vi "TUNA parse navigation string.vi"(2 "Header":string="T", 3 "Nav String":string="$,A,43,13,230,B,10,20,120,C,10,10,330,D,14,36,110,T,08,12,234\r") -> (0 "Valid?":bool, 1 "Output GPS":cluster{"X POS":i32, "Y POS":i32, "HEADING":dbl})   [LabVIEW 2014]
doc: "This VI will parse the Tug navigation string for the Tug letters, A for example, and the time, T. It returns a cluster with the Tug / Time and three values as decimals."
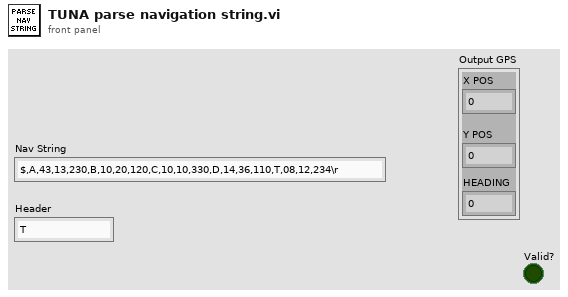
[diagram p1: front panel]
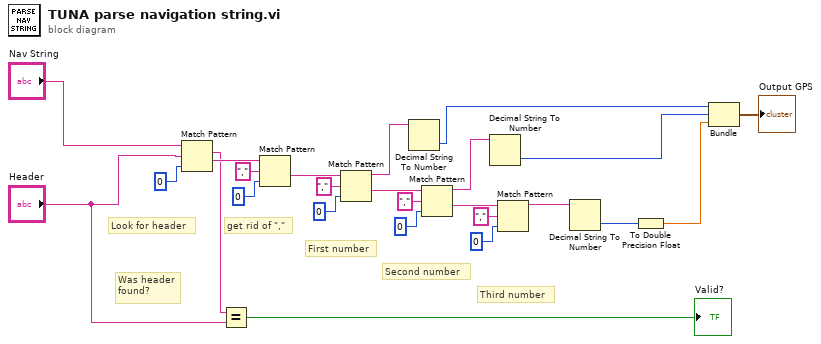
[diagram p0: block diagram]
diagram:
  # "Was header\nfound?"
  # "Third number"
  # "Second number"
  # "First number"
  # "get rid of \",\""
  # "Look for header"
  n1 = Match Pattern(string="Nav String", regular expression="Header", offset (0)=0) -> (match substring=w8:string, after substring=w10:string)  [unwired: 2 out]
  n2 = Equal?(x=w8, y="Header") -> (x = y?=→"Valid?":bool)
  n3 = Match Pattern(string=w10, regular expression=",", offset (0)=0) -> (after substring=w11:string)  [unwired: 3 out]
  n4 = Match Pattern(string=w11, regular expression=",", offset (0)=0) -> (before substring=w22:string, after substring=w18:string)  [unwired: 2 out]
  n5 = Decimal String To Number(string=w22) -> (number=w4:i32)  [unwired: 2 in, 1 out]
  n6 = Match Pattern(string=w18, regular expression=",", offset (0)=0) -> (before substring=w19:string, after substring=w14:string)  [unwired: 2 out]
  n7 = Decimal String To Number(string=w19) -> (number=w3:i32)  [unwired: 2 in, 1 out]
  n8 = Match Pattern(string=w14, regular expression=",", offset (0)=0) -> (before substring=w15:string)  [unwired: 3 out]
  n9 = Decimal String To Number(string=w15) -> (number=w2:i32)  [unwired: 2 in, 1 out]
  n10 = To Double Precision Float(number=w2) -> (double precision float=w1:dbl)
  n11 = Bundle(w4, w3, w1) -> (→"Output GPS":cluster{i32, i32, dbl})  [unwired: 1 in]
